vi "Get Matrix - file.vi"(7 "is string":bool, 8 "error in (no error)":errorcluster, 10 "variable name":string, 11 "GOLPI ref. in":T1={"pipe handle"={"lv_proc.dll file path"=path "", "process instance handle"=[]}, "fast read timeout [ms]"=500, "fast read settle time [ms]"=10, "fast read to multiple [ms]"=1, "max elements per input line"=100}) -> (0 "error out":errorcluster, 1 "cmplx double array":cdb[][](array[numeric]), 2 "double array":dbl[][](array[numeric]), 3 "GOLPI ref. out":T1={"pipe handle"={"lv_proc.dll file path"=path "", "process instance handle"=[]}, "fast read timeout [ms]"=500, "fast read settle time [ms]"=10, "fast read to multiple [ms]"=1, "max elements per input line"=100}, 5 "string array":string[](array[string]))   [LabVIEW 2013, in "GOLPI library.lvlib"]
uses:
  GOLPI library.lvlib
  Type Definitions/GOLPI reference Type Def.ctl
  LV Process.lvlibp/Pipe Handle.ctl
  Type Definitions/Custom Error Codes Enum Type Def.vi
  LV Process.lvlibp
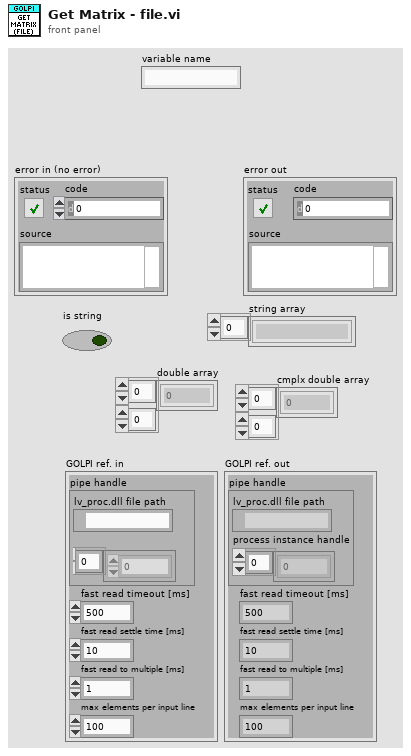
[diagram p1: front panel]
types:
  T1 = typedef "GOLPI library.lvlib/GOLPI reference Type Def.ctl" = cluster{"pipe handle":T2, "fast read timeout [ms]":u32, "fast read settle time [ms]":u32, "fast read to multiple [ms]":u32, "max elements per input line":u32}
  T2 = typedef "LV Process.lvlibp/Pipe Handle.ctl" = cluster{"lv_proc.dll file path":path, "process instance handle":u32[]}
  T3 = typedef "GOLPI library.lvlib/Custom Error Codes Enum Type Def.vi" = enum16{"no error", "00 working directory PAR1 missing", "01 octave binary PAR1 missing", "02 octave report error PAR1", "03 empty output last cmd PAR1", "04 missing temporary file PAR1", "10 var PAR1 not string", "11 var PAR1 not num, scal, ~compl", "12 var PAR1 not num, scal, compl", "13 var PAR1 not num, vect, ~compl", "14 var PAR1 not num, vect, compl", "15 var PAR1 not num, mat, ~compl", "16 var PAR1 not num, mat, ~compl", "99 not finished"}
  T4 = enum16{"open", "replace", "create", "open or create", "replace or create", "replace or create with confirmation"}
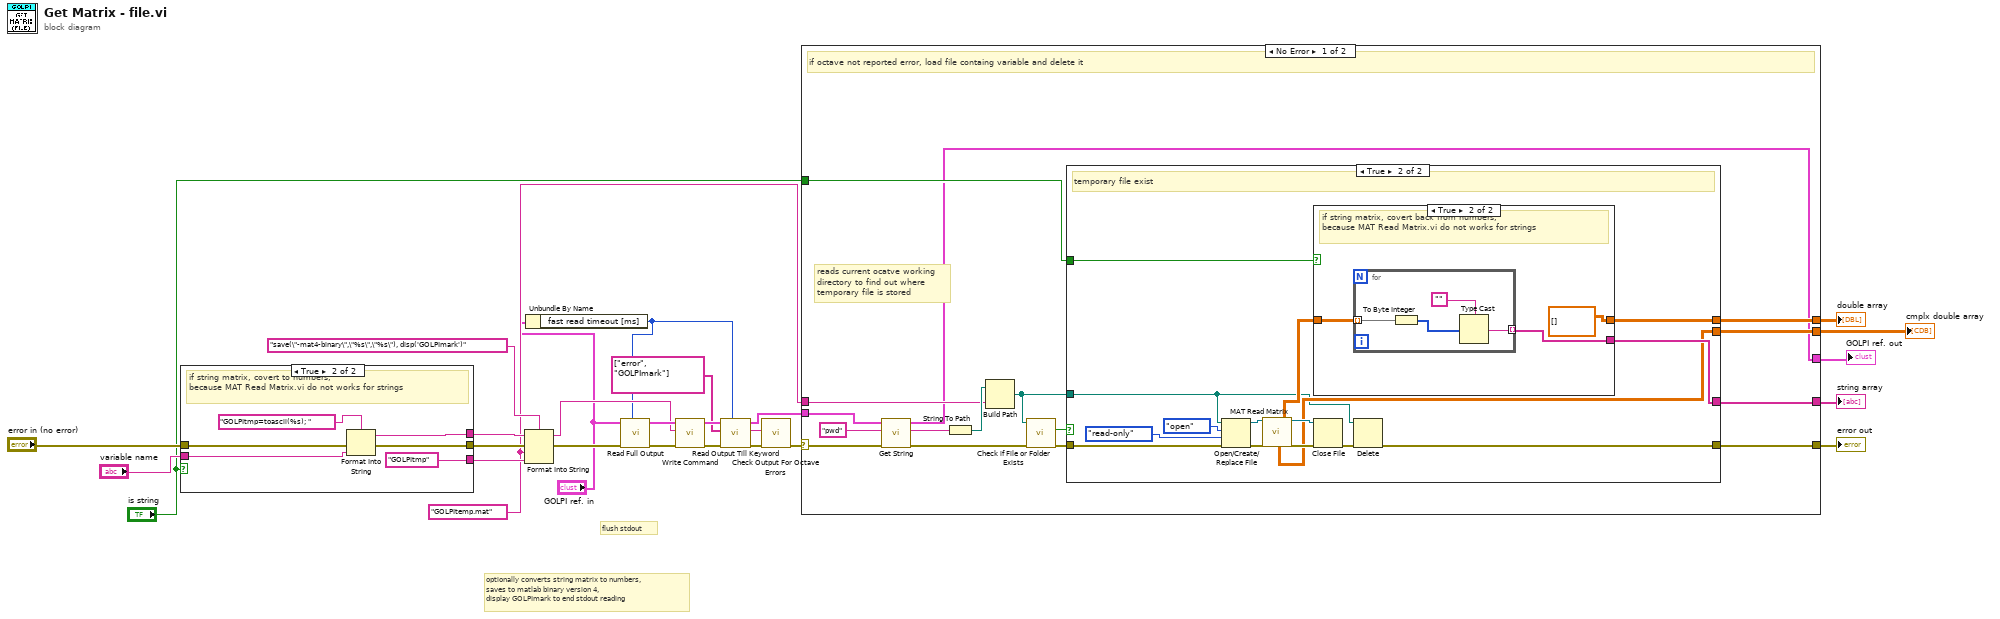
[diagram p0: block diagram]
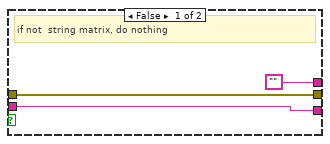
[diagram p2: hidden frame]
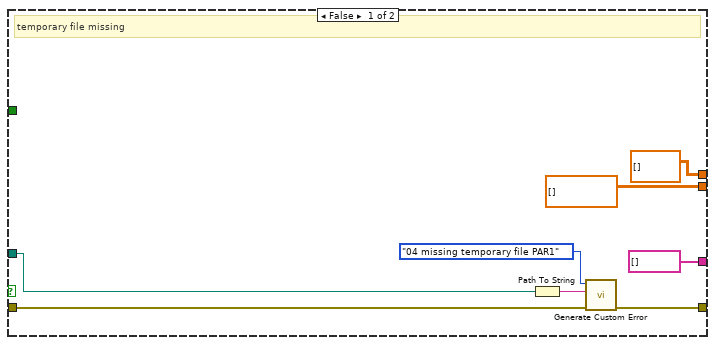
[diagram p3: hidden frame]
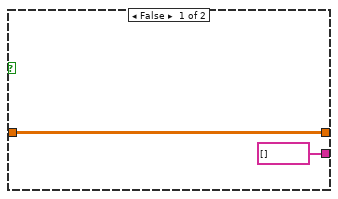
[diagram p4: hidden frame]
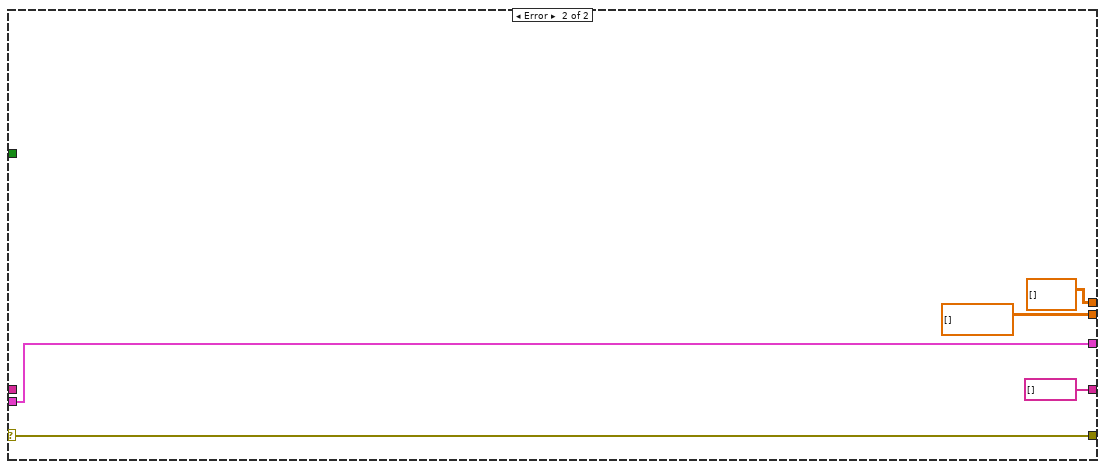
[diagram p5: hidden frame]
diagram:
  w5 = "GOLPItemp.mat" ("name or relative path")
  # "optionally converts string matrix to numbers,\nsaves to matlab binary version 4,\ndisplay GOLPImark to end stdout reading"
  # "flush stdout"
  n1 = case shown="True" "is string" {
    tunnel: ["" w34] -> w12
    tunnel: [w28 "GOLPItmp" ("format string")] -> w13
    tunnel: "variable name" -> [w28 w32]
    tunnel: [w27 w30] -> w11
    tunnel: "error in (no error)" -> [w27 w31]
    frame False {
      # "if not  string matrix, do nothing"
    }
    frame True {
      # "if string matrix, covert to numbers,\nbecause MAT Read Matrix.vi do not works for strings"
      n2 = Format Into String(format string="GOLPItmp=toascii(%s); ", error in=w31, w32) -> (resulting string=w34:string, error out=w30:errorcluster)  [unwired: 1 in]
    }
  }
  n3 = Format Into String(format string="save(\"-mat4-binary\",\"%s\",\"%s\"), disp('GOLPImark')", initial string=w12, error in=w11, w5, w13) -> (resulting string=w17:string, error out=w23:errorcluster)
  n4 = Unbundle By Name("GOLPI ref. in") -> ("fast read timeout [ms]"=w2:u32)
  n5 = call "Read Full Output.vi"("timeout [ms]"=w2, "error in"=w23, "GOLPI ref. in"="GOLPI ref. in") -> ("error out"=w24:errorcluster, "GOLPI ref. out"=w25:T1)  [unwired: 5 in, 2 out]
  n6 = call "Write Command.vi"("error in"=w24, "command"=w17, "GOLPI ref. in"=w25) -> ("error out"=w22:errorcluster, "GOLPI ref. out"=w19:T1)  [unwired: 7 in]
  n7 = call "Read Output Till Keyword.vi"("timeout [ms]"=w2, "error in"=w22, "keywords"=string[] ["error", "GOLPImark"], "GOLPI ref. in"=w19) -> ("error out"=w21:errorcluster, "read buffer"=w20:string, "GOLPI ref. out"=w4:T1)  [unwired: 4 in, 1 out]
  n8 = call "Check Output For Octave Errors.vi"("error in"=w21, "read buffer"=w20) -> ("error out"=w15:errorcluster)  [unwired: 9 in]
  n9 = case shown="No Error" w15 {
    selector: w15 -> [w41 w88]
    tunnel: [w51 w88] -> w26
    tunnel: [w49 string[] []] -> w8
    tunnel: "is string" -> [w50 _]
    tunnel: [w48 dbl[][] [] ("double array")] -> w7
    tunnel: [w47 cdb[][] [] ("CDB")] -> w6
    tunnel: w5 -> [w45 _]
    tunnel: w4 -> [w38 w84]
    tunnel: [w37 w84] -> w3
    frame No Error {
      # "reads current ocatve working\ndirectory to find out where\ntemporary file is stored"
      # "if octave not reported error, load file containg variable and delete it"
      n10 = call "Get String.vi"("error in"=w41, "variable name"="pwd", "GOLPI ref. in"=w38) -> ("error out"=w40:errorcluster, "value"=w36:string, "GOLPI ref. out"=w37:T1)  [unwired: 6 in]
      n11 = String To Path(string=w36) -> (path=w46:path)
      n12 = Build Path(base path=w46, name or relative path=w45) -> (appended path=w43:path)
      n13 = call <vilib>:"Check if File or Folder Exists.vi"("error in (no error)"=w40, "path"=w43) -> ("error out"=w44:errorcluster, "file or folder exists?"=w42:bool)  [unwired: 7 in, 1 out]
      n14 = case shown="True" w42 {
        tunnel: [w58 w67] -> w51
        tunnel: w50 -> [_ w66]
        tunnel: [string[] [] w64] -> w49
        tunnel: [dbl[][] [] ("double array") w63] -> w48
        tunnel: [cdb[][] [] ("CDB") w62] -> w47
        tunnel: w44 -> [w59 w61]
        tunnel: w43 -> [w53 w60]
        frame False {
          # "temporary file missing"
          n15 = Path To String(path=w53) -> (string=w52:string)
          n16 = call "Generate Custom Error.vi"("error in"=w59, "PAR1"=w52, "GOLPI error"=Custom_Error_Codes_Enum_Type_Def.vi."04 missing temporary file PAR1" ("Enum")) -> ("error out"=w58:errorcluster)  [unwired: 8 in]
        }
        frame True {
          # "temporary file exist"
          n17 = Open/Create/Replace File(file path (use dialog)=w60, error in=w61, operation (0:open)=T4."open", access (0:read/write)=enum16{"read/write", "read-only", "write-only"}."read-only") -> (refnum out=w71:refnum<file>, error out=w73:errorcluster)  [unwired: 2 in, 1 out]
          n18 = call "MAT Read Matrix.vi"("Ref Num"=w71, "Error In"=w73) -> ("CDB"=w62:cdb[][], "DBL"=w65:dbl[][], "Dup Ref Num"=w72:refnum<file>, "error out"=w74:errorcluster)  [unwired: 5 in, 9 out]
          n19 = case shown="True" w66 {
            tunnel: w65 -> [w75 w79]
            tunnel: [string[] [] w78] -> w64
            tunnel: [w75 dbl[][] [] ("double array")] -> w63
            frame False {
            }
            frame True {
              # "if string matrix, covert back from numbers,\nbecause MAT Read Matrix.vi do not works for strings"
              n20 = for {
                tunnel: [w83] -> w78 mode=indexing
                tunnel: w79 -> [w80] mode=indexing
                n21 = To Byte Integer(number=w80) -> (8bit integer=w81:i8[])
                n22 = Type Cast(type="", x=w81) -> (*(type *) &x=w83:string)
              }
            }
          }
          n23 = Close File(refnum=w72, error in=w74) -> (error out=w68:errorcluster)  [unwired: 1 out]
          n24 = Delete(path (use dialog)=w60, error in=w68) -> (error out=w67:errorcluster)  [unwired: 3 in, 2 out]
        }
      }
    }
    frame Error {
    }
  }
  "error out" <- w26
  "string array" <- w8
  "double array" <- w7
  "cmplx double array" <- w6
  "GOLPI ref. out" <- w3
